vi "Check if Window Name Taken.vi"(10 "windows in":T1[](array[typedef]), 11 "name":string) -> (2 "taken":bool)   [LabVIEW 2019, in "Engine Simulation Toolkit System Explorer.lvlib"]
uses:
  Engine Simulation Toolkit System Explorer.lvlib
  Event Timing Window.ctl
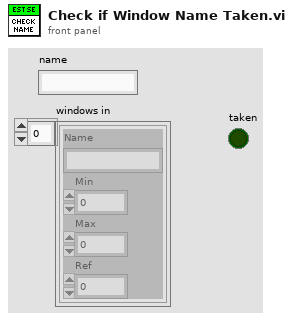
[diagram p1: front panel]
types:
  T1 = typedef "Engine Simulation Toolkit System Explorer.lvlib/Event Timing Window.ctl" = cluster{"Name":string, "Min":dbl, "Max":dbl, "Ref":dbl}
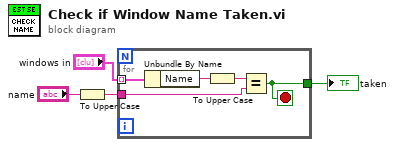
[diagram p0: block diagram]
diagram:
  n1 = To Upper Case(1:"name") -> (0:w2:string)
  n2 = for {
    tunnel: "windows in" -> [w9] mode=indexing
    tunnel: w2 -> [w6]
    tunnel: [w5] -> w1
    stop <- w5 stop-if-true
    n3 = Unbundle By Name(w9) -> ("Name"=w8:string)
    n4 = To Upper Case(1:w8) -> (0:w7:string)
    n5 = Equal?(x=w7, y=w6) -> (x = y?=w5:bool)
  }
  "taken" <- w1
